vi "Target in Stat Table.vi"(0 "Stat ID Column":string[](array[string]), 11 "Target Parameters":string) -> (4 "LastDataIndex":i32, 15 "TargetInStats":bool)   [LabVIEW 2013]
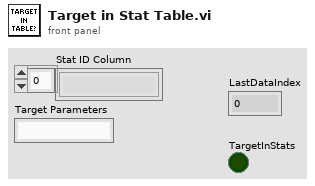
[diagram p1: front panel]
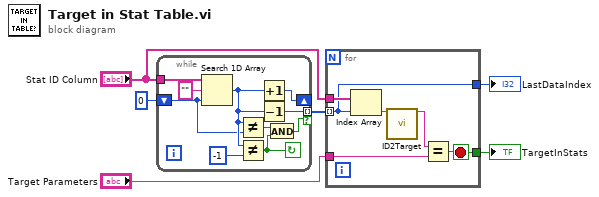
[diagram p0: block diagram]
diagram:
  n1 = while {
    tunnel: "Stat ID Column" -> [w16]
    shift-right: [w11] -> _
    shift-left: 0 ("index of element") -> [w10]
    tunnel: [w13] -> w6 mode=indexing if=w7
    stop <- w8 continue-if-true
    n2 = Search 1D Array(1D array=w16, element="", start index (0)=w10) -> (index of element=w12:i32)
    n3 = Not Equal?(x=w12, y=w10) -> (x != y?=w9:bool)
    n4 = Not Equal?(x=w12, y=-1) -> (x != y?=w8:bool)
    n5 = Increment(x=w12) -> (x+1=w11:i32)
    n6 = Decrement(x=w12) -> (x-1=w13:i32)
    n7 = And(x=w9, y=w8) -> (x .and. y?=w7:bool)
  }
  n8 = for {
    tunnel: w6 -> [w17] mode=indexing
    tunnel: "Stat ID Column" -> [w22]
    tunnel: "Target Parameters" -> [w19]
    tunnel: [w18] -> w2
    tunnel: [w17] -> w1
    stop <- w18 stop-if-true
    n9 = Index Array(array=w22, index=w17) -> (element=w21:string)
    n10 = call "ID2Target.vi"("UniqueID"=w21) -> ("Target Parameters"=w20:string)  [unwired: 13 in, 1 out]
    n11 = Equal?(x=w20, y=w19) -> (x = y?=w18:bool)
  }
  "TargetInStats" <- w2
  "LastDataIndex" <- w1
